vi "getLinkedNodes.vi"(8 "error in (no error)":errorcluster, 11 "GraphNode in":refnum<class "GraphNode.lvclass">) -> (0 "error out":errorcluster, 2 "LinkedNodes":refnum<data-value>[](array[refnum]), 3 "GraphNode out":refnum<class "GraphNode.lvclass">)   [LabVIEW 2010, in "GraphNode.lvclass"]
uses:
  GraphNode.lvclass
  GraphNode.lvclass/GraphNode.ctl
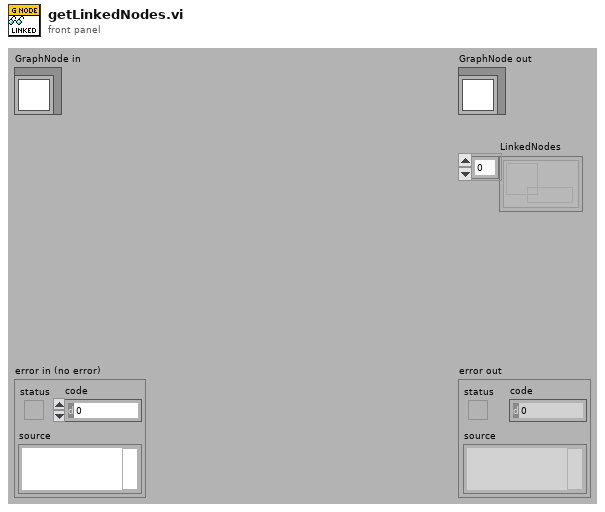
[diagram p1: front panel]
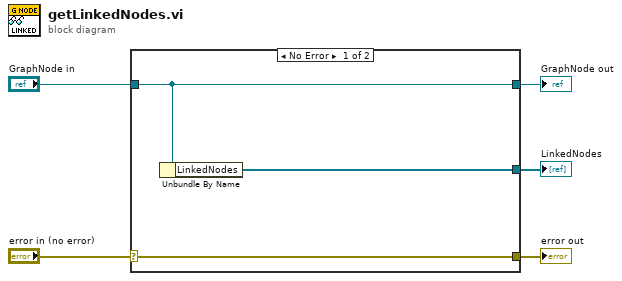
[diagram p0: block diagram]
diagram:
  n1 = case shown="No Error" "error in (no error)" {
    selector: "error in (no error)" -> [w8 w9]
    tunnel: [w8 w9] -> w4
    tunnel: [w7 w10] -> w2
    tunnel: "GraphNode in" -> [w7 w10]
    tunnel: [w6 _] -> w1
    frame No Error {
      n2 = Unbundle By Name(w7) -> ("LinkedNodes"=w6:refnum<data-value>[])
    }
    frame Error {
    }
  }
  "error out" <- w4
  "GraphNode out" <- w2
  "LinkedNodes" <- w1
